vi "niRFUtil WFM Remove Origin Offset.vi"(0 "Signal In":T1 {"y" format="%.2f"; "dx" format="%^.2e"; "x0" format="%^.2e"}, 2 "Remove? (T)":bool=TRUE, 5 "Reference Signal In":T1 {"y" format="%.2f"; "dx" format="%^.2e"; "x0" format="%^.2e"}) -> (4 "Signal Out":T1 {"y" format="%.2f"; "dx" format="%^.2e"; "x0" format="%^.2e"}, 6 "Reference Signal Out":T1 {"y" format="%.2f"; "dx" format="%^.2e"; "x0" format="%^.2e"}, 13 "Origin Offset, dBc":sgl format="%.2f", 14 "Origin Offset":csg format="%.3f")   [LabVIEW 2015, in "niRFUtil.lvlib"]
doc: "(c) Copyright 2006, National Instruments, Inc. This VI may not be duplicated, sold, or distributed without written consent from National Instruments."
uses:
  niRFUtil.lvlib
  Includes/niRFUtil INC Complex Waveform.ctl
  Includes/niRFUtil INC Complex Array.ctl
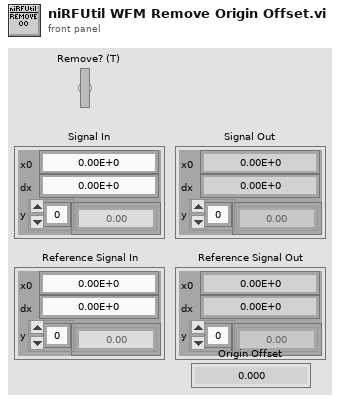
[diagram p1: front panel]
types:
  T1 = typedef "niRFUtil.lvlib/niRFUtil INC Complex Waveform.ctl" = cluster{"x0":dbl, "dx":dbl, "y":T2}
  T2 = typedef "niRFUtil.lvlib/niRFUtil INC Complex Array.ctl" = csg[]
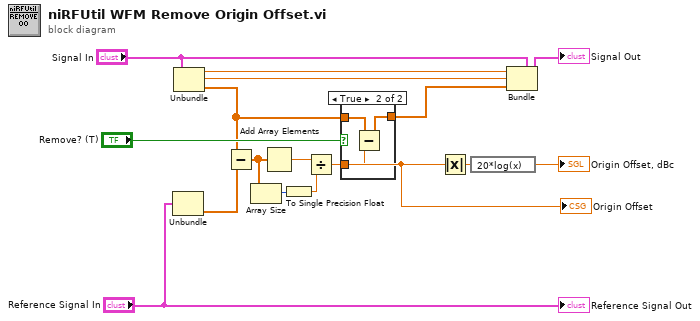
[diagram p0: block diagram]
diagram:
  n1 = Unbundle("Reference Signal In") -> ("y"=w10:T2)  [unwired: 2 out]
  n2 = Unbundle("Signal In") -> ("x0"=w8:dbl, "dx"=w7:dbl, "y"=w3:T2)
  n3 = Subtract(x=w3, y=w10) -> (x-y=w13:T2)
  n4 = Array Size(array=w13) -> (size(s)=w11:i32)
  n5 = Add Array Elements(numeric array=w13) -> (sum=w12:csg)
  n6 = To Single Precision Float(number=w11) -> (single precision float=w1:sgl)
  n7 = Divide(x=w12, y=w1) -> (x/y=w6:csg)
  "Origin Offset" <- w6
  n8 = case shown="True" "Remove? (T)" {
    tunnel: w6 -> [_ w20]
    tunnel: w3 -> [w17 w19]
    tunnel: [w17 w18] -> w2
    frame False {
    }
    frame True {
      n9 = Subtract(x=w19, y=w20) -> (x-y=w18:T2)
    }
  }
  n10 = Absolute Value(x=w6) -> (abs(x)=w14:sgl)
  n11 = expression code="20*log(x)"(w14) -> (→"Origin Offset, dBc":sgl)
  n12 = Bundle(cluster="Signal In", "x0"=w8, "dx"=w7, "y"=w2) -> (→"Signal Out":T1)
  "Reference Signal Out" <- "Reference Signal In"
